vi "Read Data.vi"(8 "error in":errorcluster, 11 "AlicatVData in":refnum<class "AlicatVCData.lvclass">) -> (0 "error out":errorcluster, 1 "sp":sgl, 2 "val":sgl, 3 "AlicatVData out":refnum<class "AlicatVCData.lvclass">)   [LabVIEW 2014, in "Alicat.lvlib" / "AlicatVCData.lvclass"]
uses:
  AlicatVCData.lvclass
  AlicatVCData.lvclass/AlicatVCData.ctl
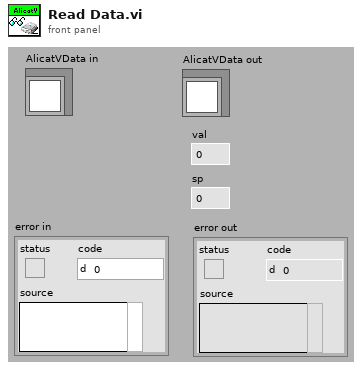
[diagram p1: front panel]
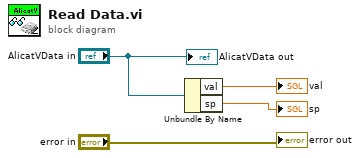
[diagram p0: block diagram]
diagram:
  n1 = Unbundle By Name("AlicatVData in") -> ("val"=→"val":sgl, "sp"=→"sp":sgl)
  "error out" <- "error in"
  "AlicatVData out" <- "AlicatVData in"
